vi "2.vi"(8 "Error In":errorcluster, 10 "Array":bool[](array[boolean]), 11 "buffer in":cluster{"PIPE IN":i32, "PIPE OUT":i32}) -> (0 "Error Out":errorcluster, 3 "buffer out":cluster{"PIPE IN":i32, "PIPE OUT":i32})   [LabVIEW 2016]
uses:
  microchip_solutions_v2013-06-15/USB/Tools/MCHPUSB Custom Driver/Mpusbapi/Dll/Borland_C/Source/mpusbapi.dll
panel:
  out "pLength":i32
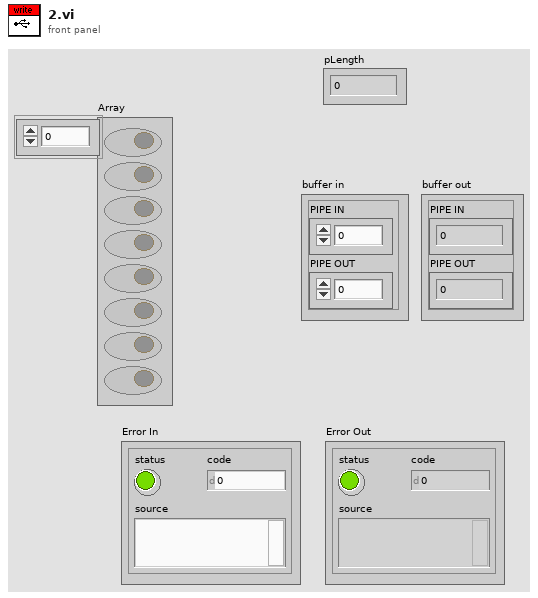
[diagram p1: front panel]
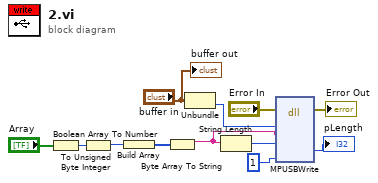
[diagram p0: block diagram]
diagram:
  n1 = Boolean Array To Number(Boolean array="Array") -> (number=w11:u32)
  n2 = To Unsigned Byte Integer(number=w11) -> (unsigned 8bit integer=w9:u8)
  n3 = Build Array(w9) -> (w10:u8[])
  n4 = Byte Array To String(unsigned byte array=w10) -> (string=w8:string)
  n5 = Unbundle("buffer in") -> ("PIPE OUT"=w4:i32)  [unwired: 1 out]
  n6 = String Length(string=w8) -> (length=w7:i32)
  n7 = dll-call lib="C:/microchip_solutions_v2013-06-15/USB/Tools/MCHPUSB Custom Driver/Mpusbapi/Dll/Borland_C/Source/mpusbapi.dll" fn="MPUSBWrite"(error in="Error In", "PIPE OUT"=w4, "pData"=w8, "dwlen"=w7, "dwMilliseconds"=1) -> (error out=→"Error Out":errorcluster, "pLength"=→"pLength":i32)  [unwired: 8 in, 1 out]
  "buffer out" <- "buffer in"
